vi "Get Object Refs from Node.vi"(8 "error in (no error)":errorcluster, 11 "Data Value Reference in":T2) -> (0 "error out":errorcluster, 3 "object Refs":T1)   [LabVIEW 2013, in "Modbus Module editor node.lvclass"]
uses:
  Modbus Module editor node.lvclass
  <vilib>/NI/Configuration Framework/Node/NodeRef.ctl
  <vilib>/NI/Configuration Framework/Node/NISE_CEF_Node.lvclass
  <vilib>/NI/DCAF Table API/Table Manager/object ref.ctl
  <vilib>/NI/DCAF/Tag Editor Core/Configuration Editor/Classes/Engine Parent/Engine Parent Editor Node.lvclass
  <vilib>/NI/DCAF/Tag Editor Core/Configuration Editor/Classes/Module editor node/module editor node.lvclass
  <vilib>/NI/DCAF Table API/Table Manager/Table Manager.lvclass
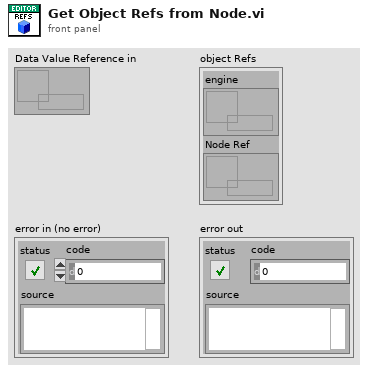
[diagram p1: front panel]
types:
  T1 = typedef "Table Manager.lvlib/Table Manager.lvclass/object ref.ctl" = cluster{"engine":refnum<data-value>, "Node Ref":refnum<data-value>}
  T2 = typedef "NISE_CEF_Node.lvclass/NodeRef.ctl" = refnum<data-value>
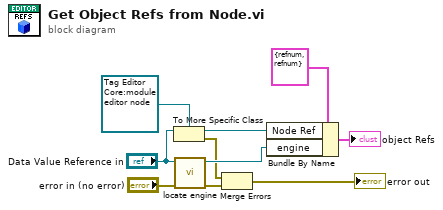
[diagram p0: block diagram]
diagram:
  n1 = To More Specific Class(target class=refnum<data-value> refnum ("data value reference"), reference="Data Value Reference in") -> (specific class reference=w8:refnum<data-value>, error out=w2:errorcluster)  [unwired: 1 in]
  n2 = call <vilib>:"locate engine.vi"("error in"="error in (no error)", "component"="Data Value Reference in") -> ("error out"=w3:errorcluster, "engine"=w7:refnum<data-value>)  [unwired: 8 in]
  n3 = Merge Errors(w2, w3) -> (→"error out":errorcluster)
  n4 = Bundle By Name(cluster=T1 {"engine"=refnum, "Node Ref"=refnum} ("object refs"), "Node Ref"=w8, "engine"=w7) -> (→"object Refs":T1)
